vi "PTScanner.add step obj.vi"(0 "array":T1[](array[typedef]), 2 "obj index":i32, 4 "nomValue":dbl) -> (14 "appended array":T1[](array[typedef]))   [LabVIEW 2014, in "PTScanner.lvlib"]
uses:
  PTScanner.lvlib
  PTScanner.step obj parameters.ctl
panel:
  in  "step obj params":T1
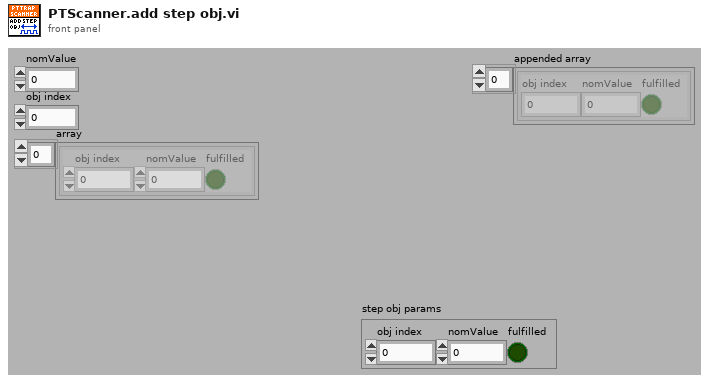
[diagram p1: front panel]
types:
  T1 = typedef "PTScanner.lvlib/PTScanner.step obj parameters.ctl" = cluster{"obj index":i32, "nomValue":dbl, "fulfilled":bool}
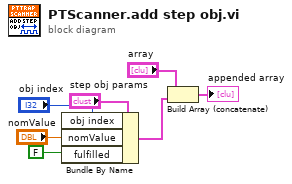
[diagram p0: block diagram]
diagram:
  n1 = Bundle By Name(cluster="step obj params", "obj index"="obj index", "nomValue"="nomValue", "fulfilled"=FALSE) -> (w7:T1)
  n2 = Build Array (concatenate)("array", w7) -> (→"appended array":T1[])
